vi "SetStationFullName.vi"(8 "error in":errorcluster, 10 "StationFullName":string, 11 "SequenceRun in":refnum<class "SequenceRun.lvclass">) -> (0 "error out":errorcluster, 3 "SequenceRun out":refnum<class "SequenceRun.lvclass">)   [LabVIEW 2021, in "ProligentXMLGenerator.lvlib" / "SequenceRun.lvclass"]
doc: "Defines the name the product for the current process run.\n\"[Root Station/][[Path/]...]Name\"\nEach path strings and the name are limited to 64 characters and the total string provided is limited to 2000 characters.\n\nWARNING:\n\nSince the '/' character is the hierarchy delimiter, if a path string contains a '/' character it will be interpreted as\na new hierarchy. It is therefore suggested to replace '/' by '-' in all your path components to keep the expected hierarchy.\nFor example, if you have a sequence named 'PASS/FAIL' and you don't substitude '/' by '-', the 'PASS' would be interpreted \nas a sequence category while 'FAIL' would be the name of a sequence. If you do the suggested substitution, the name of \nthe sequence would be interpreted as 'PASS-FAIL' without any category."
uses:
  SequenceRun.lvclass
  SequenceRun.lvclass/SequenceRun.ctl
  Base/FullName/FullName.lvclass
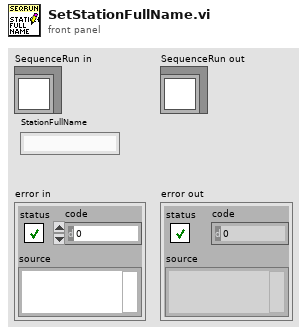
[diagram p1: front panel]
types:
  T1 = typedef "ProligentXMLGenerator.lvlib/SequenceRun.lvclass/Data.ctl" = cluster{"Name":string, "StepRuns":refnum<class "StepRun.lvclass">[], "Characteristics":refnum<class "Characteristic.lvclass">[], "Documents":refnum<class "Document.lvclass">[], "FailureReferences":refnum<class "FailureReference.lvclass">[], "CustomData":refnum<class "CustomData.lvclass">, "StartDate":refnum<class "DateTime.lvclass">, "EndDate":refnum<class "DateTime.lvclass">, "SequenceExecutionStatus":refnum<class "ExecutionStatus.lvclass">, "SequenceRunId":refnum<class "Guid.lvclass">, "SequenceFullName":refnum<class "SequenceFullName.lvclass">, "SequenceVersion":refnum<class "NonEmptyString_64.lvclass">, "StationFullName":refnum<class "FullName.lvclass">, "User":refnum<class "NonEmptyString_255.lvclass">, "TimeZoneInfoId":string}
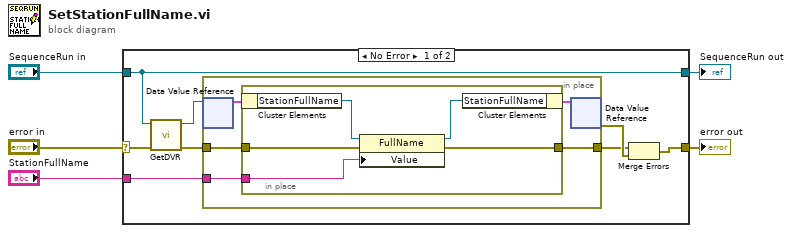
[diagram p0: block diagram]
diagram:
  n1 = case shown="No Error" "error in" {
    selector: "error in" -> [w11 w24]
    tunnel: "SequenceRun in" -> [w6 w25]
    tunnel: [w8 w24] -> w3
    tunnel: "StationFullName" -> [w7 _]
    tunnel: [w6 w25] -> w1
    frame No Error {
      n2 = call "GetDVR.vi"("error in"=w11, "SequenceRun"=w6) -> ("error out"=w10:errorcluster, "DVRReference"=w12:refnum<data-value>)  [unwired: 8 in]
      n3 = in-place "In Place Element Structure" {
        in-place-border: w10 -> [w18]
        in-place-border: [w17] -> w9
        in-place-border: w7 -> [w16]
        n4 = in-place-dvr #1(w12) -> (w15:T1)  [unwired: 1 out]
        n5 = in-place "In Place Element Structure" {
          in-place-border: w18 -> [w23]
          in-place-border: [w22] -> w17
          in-place-border: w16 -> [w21]
          n6 = in-place-cluster #2(w15) -> ("StationFullName"=w20:refnum<class "FullName.lvclass">)
          n7 = property on="Property Node" class="FullName"(reference=w20, error in=w23, "Value"=w21) -> (reference out=w19:refnum<class "FullName.lvclass">, error out=w22:errorcluster)
          n8 = in-place-cluster #2("StationFullName"=w19) -> (w14:T1)
        }
        n9 = in-place-dvr #1(w14) -> (w13:errorcluster)  [unwired: 1 out]
      }
      n10 = Merge Errors(w9, w13) -> (w8:errorcluster)
    }
    frame Error {
    }
  }
  "error out" <- w3
  "SequenceRun out" <- w1
